vi "Aux TE Controllers Runtime.vi"(8 "Error In":errorcluster, 9 "TE Serial Ports In":T4[](array[typedef]) {"XOFF Char" format="%.0x"; "XON Char" format="%.0x"; "flow control" items=["None"=0, "XON/XOFF"=1, "RTS/CTS"=2, "DTR/DSR"=4]; "stop bits" items=["1.0"=10, "1.5"=15, "2.0"=20]; "data bits" min=5 max=8 step=1; "baud rate" items=["75"=75, "110"=110, "134"=134, "150"=150, "300"=300, "600"=600, "1200"=1200, "1800"=1800, "2400"=2400, "4800"=4800, "7200"=7200, "9600"=9600, "14400"=14400, "19200"=19200, "28800"=28800, "38400"=38400, "56000"=56000, "57600"=57600, "115200"=115200, "128000"=128000, "230400"=230400]; "termination char" format="%.0x"}, 10 "CmdsToWrite":string[](array[string]), 11 "Refs":T1 {"Current Settings"."Pump" items=["Pump 0", "Pump 1", "Pump 2", "Pump 3", "Pump 4", "Pump 5"]; "Current Settings"."Chart X axis Timescale" min=20 max=180 step=1; "Current Settings"."RunTime Mode Settings"."Exp. Gas Tank" items=["0.07", "0.031", "0.877", "1.863", "3.881", "5.790", "7.688", "6.000"]; "Current Settings"."RunTime Mode Settings"."Insp. Gas Tank" items=["0.07", "0.031", "0.877", "1.863", "3.881", "5.790", "7.688", "6.000"]; "Current Settings"."RunTime Mode Settings"."I:E Ratio" max=30 scale=0.0..7.0; "Current Settings"."RunTime Mode Settings"."Resp Rate Brpm" min=0 max=30 format="%.2f"; "Current Settings"."TE#2 Configuration"."Serial Port"."XOFF Char" format="%.0x"; "Current Settings"."TE#2 Configuration"."Serial Port"."XON Char" format="%.0x"; "Current Settings"."TE#2 Configuration"."Serial Port"."flow control" items=["None"=0, "XON/XOFF"=1, "RTS/CTS"=2, "DTR/DSR"=4]; "Current Settings"."TE#2 Configuration"."Serial Port"."stop bits" items=["1.0"=10, "1.5"=15, "2.0"=20]; "Current Settings"."TE#2 Configuration"."Serial Port"."data bits" min=5 max=8 step=1; "Current Settings"."TE#2 Configuration"."Serial Port"."baud rate" items=["75"=75, "110"=110, "134"=134, "150"=150, "300"=300, "600"=600, "1200"=1200, "1800"=1800, "2400"=2400, "4800"=4800, "7200"=7200, "9600"=9600, "14400"=14400, "19200"=19200, "28800"=28800, "38400"=38400, "56000"=56000, "57600"=57600, "115200"=115200, "128000"=128000, "230400"=230400]; "Current Settings"."TE#2 Configuration"."Serial Port"."termination char" format="%.0x"; "Current Settings"."TE#1 Configuration"."Serial Port"."XOFF Char" format="%.0x"; "Current Settings"."TE#1 Configuration"."Serial Port"."XON Char" format="%.0x"; "Current Settings"."TE#1 Configuration"."Serial Port"."flow control" items=["None"=0, "XON/XOFF"=1, "RTS/CTS"=2, "DTR/DSR"=4]; "Current Settings"."TE#1 Configuration"."Serial Port"."stop bits" items=["1.0"=10, "1.5"=15, "2.0"=20]; "Current Settings"."TE#1 Configuration"."Serial Port"."data bits" min=5 max=8 step=1; "Current Settings"."TE#1 Configuration"."Serial Port"."baud rate" items=["75"=75, "110"=110, "134"=134, "150"=150, "300"=300, "600"=600, "1200"=1200, "1800"=1800, "2400"=2400, "4800"=4800, "7200"=7200, "9600"=9600, "14400"=14400, "19200"=19200, "28800"=28800, "38400"=38400, "56000"=56000, "57600"=57600, "115200"=115200, "128000"=128000, "230400"=230400]; "Current Settings"."TE#1 Configuration"."Serial Port"."termination char" format="%.0x"; "Current Settings"."Capnometer Configuration"."Device" items=["None", "TidalWave", "LoFlow / Canary", "Capnogard"]; "Current Settings"."Capnometer Configuration"."Serial Port"."XOFF Char" format="%.0x"; "Current Settings"."Capnometer Configuration"."Serial Port"."XON Char" format="%.0x"; "Current Settings"."Capnometer Configuration"."Serial Port"."flow control" items=["None"=0, "XON/XOFF"=1, "RTS/CTS"=2, "DTR/DSR"=4]; "Current Settings"."Capnometer Configuration"."Serial Port"."stop bits" items=["1.0"=10, "1.5"=15, "2.0"=20]; "Current Settings"."Capnometer Configuration"."Serial Port"."data bits" min=5 max=8 step=1; "Current Settings"."Capnometer Configuration"."Serial Port"."baud rate" items=["75"=75, "110"=110, "134"=134, "150"=150, "300"=300, "600"=600, "1200"=1200, "1800"=1800, "2400"=2400, "4800"=4800, "7200"=7200, "9600"=9600, "14400"=14400, "19200"=19200, "28800"=28800, "38400"=38400, "56000"=56000, "57600"=57600, "115200"=115200, "128000"=128000, "230400"=230400]; "Current Settings"."Capnometer Configuration"."Serial Port"."termination char" format="%.0x"; "Current Settings"."DAQx Settings"."Analog Output Settings (Volts)" format="%#.3g"; "Current Settings"."DAQx Settings"."Duty Cycle" min=10.0 max=90.0 format="%.1g"; "Current Settings"."DAQx Settings"."Frequency" min=20.0 max=200.0; "Current Settings"."DataLogging Settings"."Data File Duration (Minutes)" min=2 max=200 format="%#.2g"; "Current Settings"."Calibration Settings"."Tolerance #2" min=2 max=4096; "Current Settings"."Calibration Settings"."Cal. Average" min=2 max=4096; "Current Settings"."Test Settings"."Test Sensor ID" items=["(select)", "RB", "YC", "", "Other"]}) -> (0 "Error Out":errorcluster, 1 "Read Array":string[][](array[string]), 2 "ReadData":sgl[][](array[numeric]) format="%.2g", 3 "TE Serial Ports Out":T4[](array[typedef]) {"XOFF Char" format="%.0x"; "XON Char" format="%.0x"; "flow control" items=["None"=0, "XON/XOFF"=1, "RTS/CTS"=2, "DTR/DSR"=4]; "stop bits" items=["1.0"=10, "1.5"=15, "2.0"=20]; "data bits" min=5 max=8 step=1; "baud rate" items=["75"=75, "110"=110, "134"=134, "150"=150, "300"=300, "600"=600, "1200"=1200, "1800"=1800, "2400"=2400, "4800"=4800, "7200"=7200, "9600"=9600, "14400"=14400, "19200"=19200, "28800"=28800, "38400"=38400, "56000"=56000, "57600"=57600, "115200"=115200, "128000"=128000, "230400"=230400]; "termination char" format="%.0x"}, 4 "TE Bytes Read":i16[][](array[numeric]), 5 "Set Point Good":bool, 6 "TE Data":sgl[][](array[numeric]), 7 "Set Point Disabled":bool)   [LabVIEW 2016]
uses:
  Controls/Serial Visa Control.ctl
  Controls/DAQ Needed.ctl
  Controls/Processed Variables.ctl
  Controls/AirPump Controls.ctl
  Controls/IE Ratio knob.ctl
  Controls/UI Settings.ctl
  Controls/Aux CO2 Control.ctl
  Controls/Aux CO2 Selector.ctl
  Controls/Aux TE Control.ctl
  Controls/Queues And Others.ctl
  Controls/SerialPortControl.ctl
  Miscellaneous/Globals.vi
panel:
  out "after substring":string
  out "appended array":string[][](array[string])
  out "subarray":dbl[](array[numeric])
  out "size(s)":i32[](array[numeric])
  # "Note: Setting Brpm to zero will\ndisable Insp / Exp digital output."
  # "mmHg"
  # "pts"
  # "tolerance"
  # "AN5 (Temp 1)"
  # "AN6 (Temp 2)"
  # "AN7 (Temp 3)"
  # "AN8 (T FET)"
  # "AN0 (T POT)"
  # "Tref (Set Pt))"
  # "(Spare)"
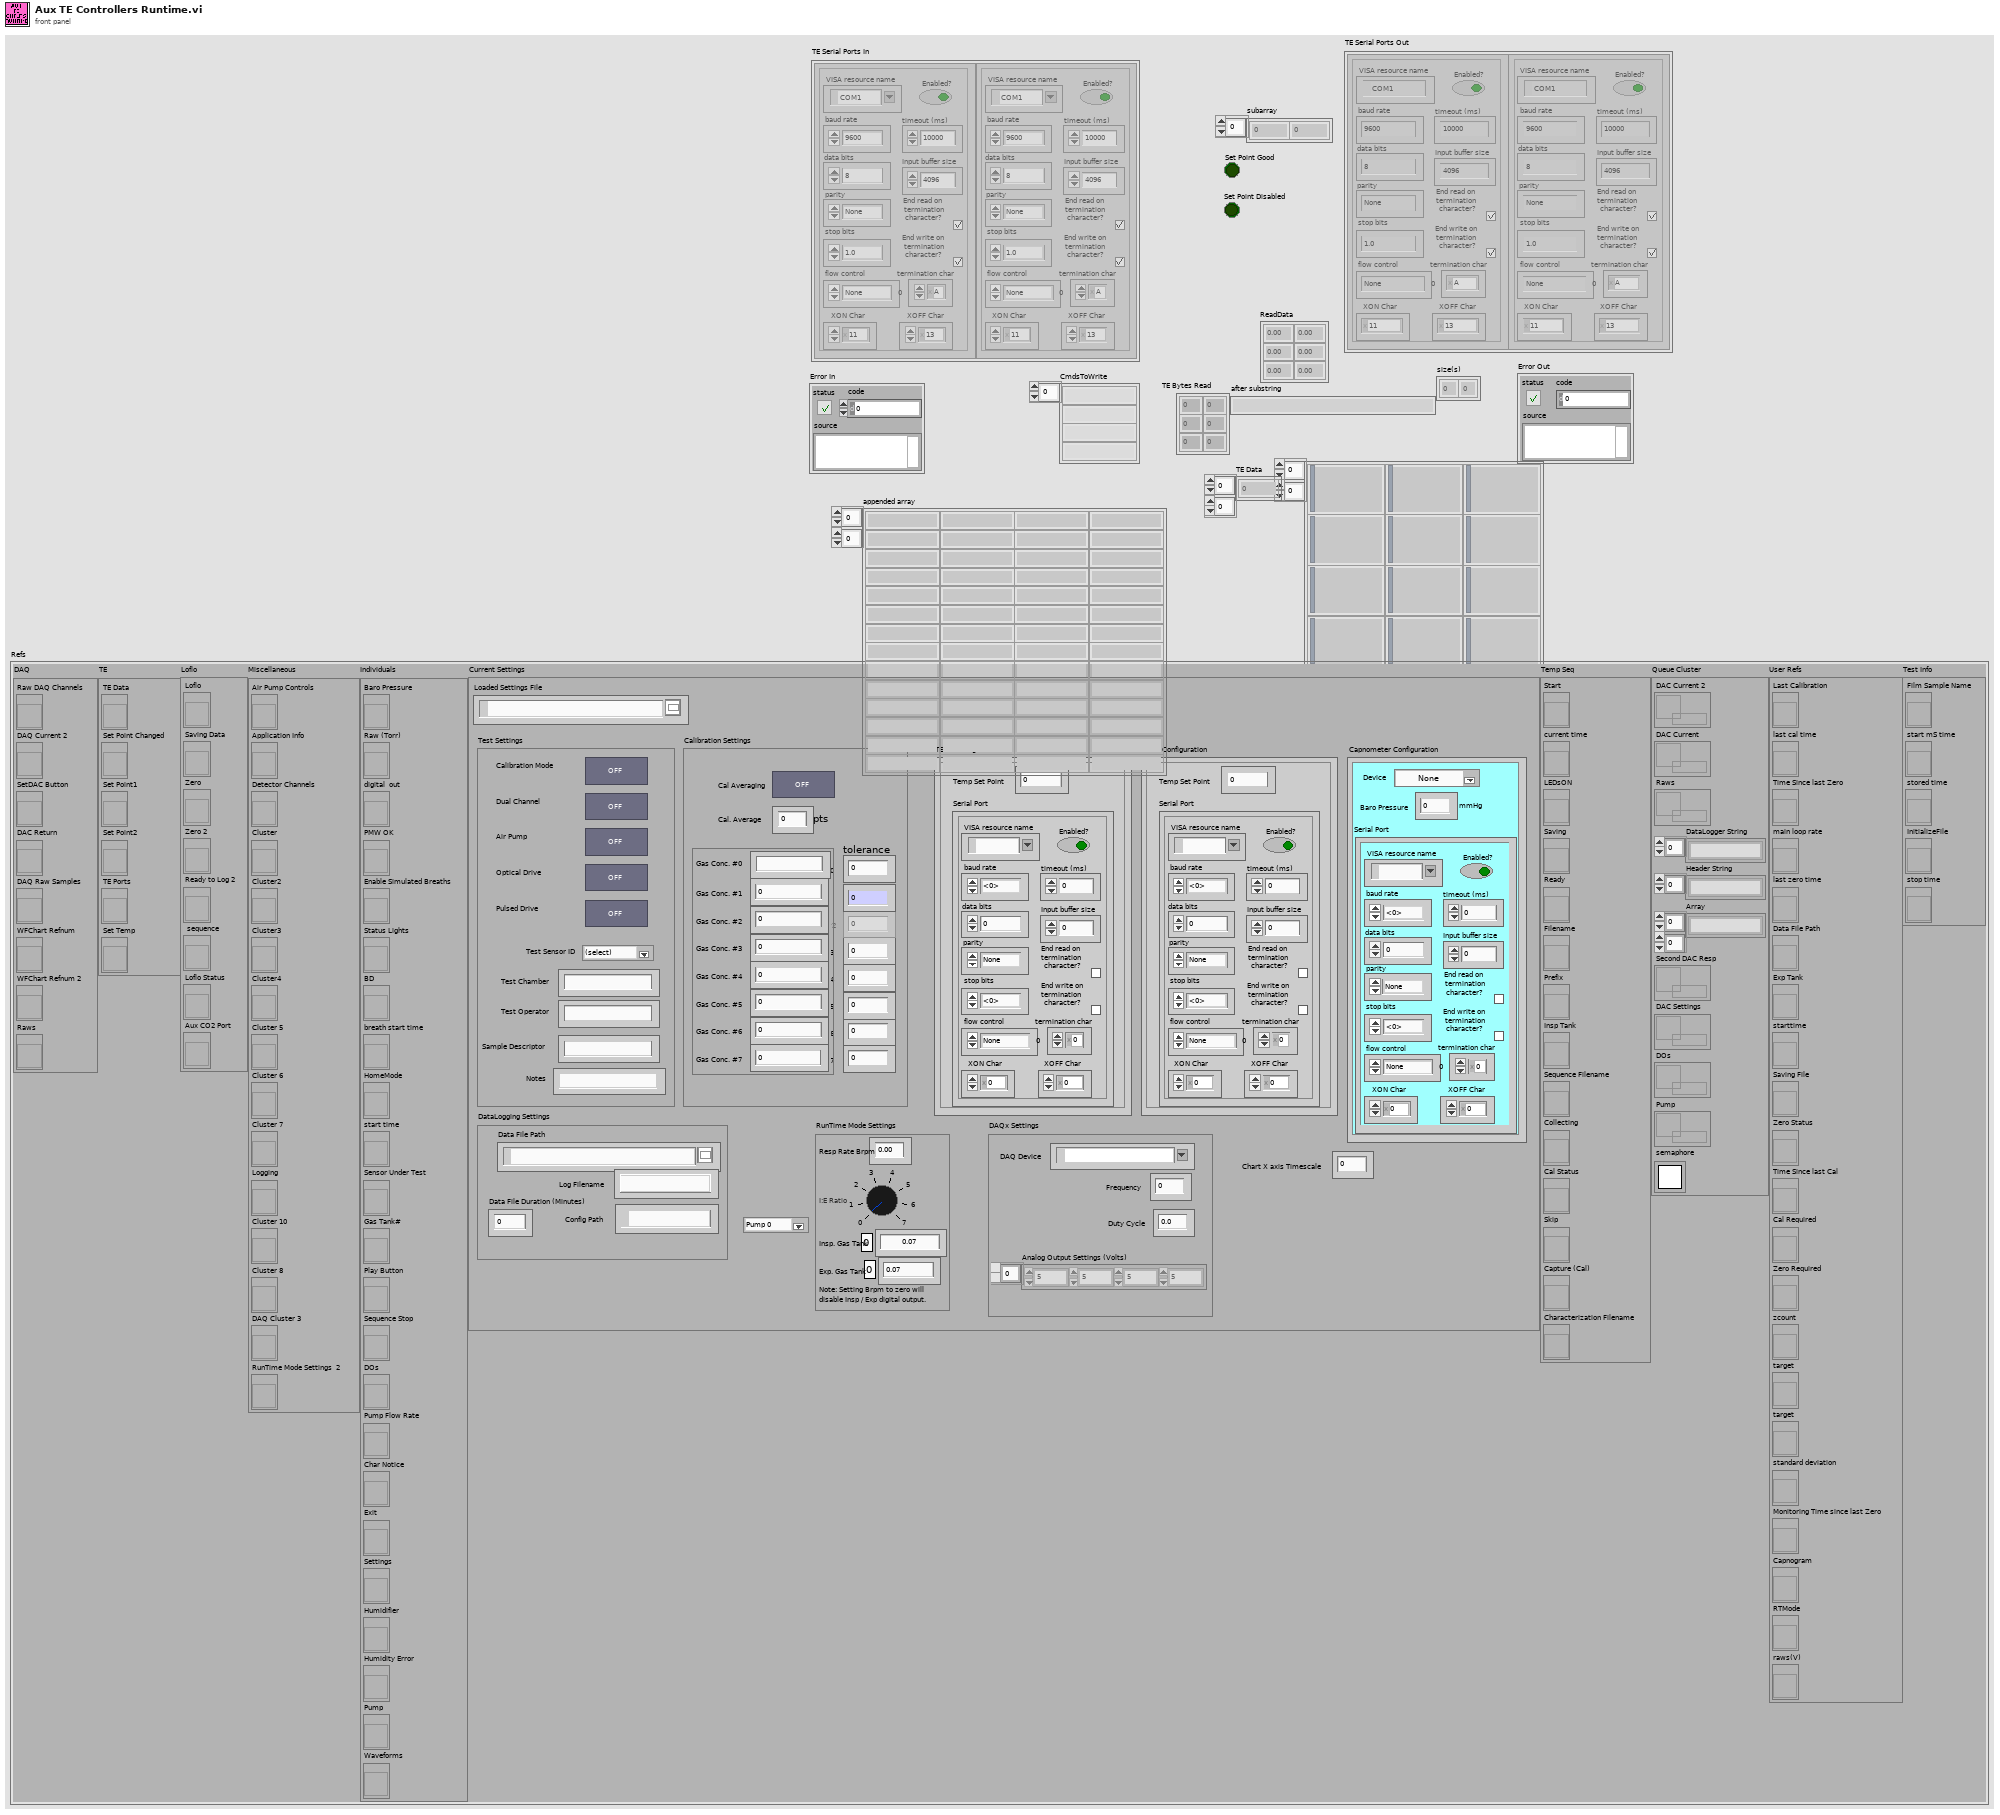
[diagram p1: front panel]
types:
  T1 = typedef "DAQ Needed.ctl" = cluster{"DAQ":cluster{"Raw DAQ Channels":refnum<vi>, "DAQ Current 2":refnum<vi>, "SetDAC Button":refnum<vi>, "DAC Return":refnum<vi>, "DAQ Raw Samples":refnum<vi>, "WFChart Refnum":refnum<vi>, "WFChart Refnum 2":refnum<vi>, "Raws":refnum<vi>}, "TE":cluster{"TE Data":refnum<vi>, "Set Point Changed":refnum<vi>, "Set Point1":refnum<vi>, "Set Point2":refnum<vi>, "TE Ports":refnum<vi>, "Set Temp":refnum<vi>}, "Loflo":cluster{"Loflo":refnum<vi>, "Saving Data":refnum<vi>, "Zero":refnum<vi>, "Zero 2":refnum<vi>, "Ready to Log 2":refnum<vi>, " sequence":refnum<vi>, "Loflo Status ":refnum<vi>, "Aux CO2 Port":refnum<vi>}, "Miscellaneous":cluster{"Air Pump Controls":refnum<vi>, "Application Info":refnum<vi>, "Detector Channels ":refnum<vi>, "Cluster":refnum<vi>, "Cluster2":refnum<vi>, "Cluster3":refnum<vi>, "Cluster4":refnum<vi>, "Cluster 5":refnum<vi>, "Cluster 6":refnum<vi>, "Cluster 7":refnum<vi>, "Logging":refnum<vi>, "Cluster 10":refnum<vi>, "Cluster 8":refnum<vi>, "DAQ Cluster 3":refnum<vi>, "RunTime Mode Settings  2":refnum<vi>}, "Individuals":cluster{"Baro Pressure":refnum<vi>, "Raw (Torr)":refnum<vi>, "digital  out":refnum<vi>, "PMW OK":refnum<vi>, "Enable Simulated Breaths":refnum<vi>, "Status Lights":refnum<vi>, "BD":refnum<vi>, "breath start time":refnum<vi>, "HomeMode":refnum<vi>, "start time":refnum<vi>, "Sensor Under Test":refnum<vi>, "Gas Tank#":refnum<vi>, "Play Button":refnum<vi>, "Sequence Stop":refnum<vi>, "DOs":refnum<vi>, "Pump Flow Rate":refnum<vi>, "Char Notice":refnum<vi>, "Exit":refnum<vi>, "Settings":refnum<vi>, "Humidifier":refnum<vi>, "Humidity Error":refnum<vi>, "Pump":refnum<vi>, "Waveforms":refnum<vi>}, "Current Settings":T2, "Temp Seq":cluster{"Start":refnum<vi>, "current time":refnum<vi>, "LEDsON":refnum<vi>, "Saving":refnum<vi>, "Ready":refnum<vi>, "Filename":refnum<vi>, "Prefix":refnum<vi>, "Insp Tank":refnum<vi>, "Sequence Filename":refnum<vi>, "Collecting":refnum<vi>, "Cal Status":refnum<vi>, "Skip":refnum<vi>, "Capture (Cal)":refnum<vi>, "Characterization Filename":refnum<vi>}, "Queue Cluster":T7, "User Refs":cluster{"Last Calibration":refnum<vi>, "last cal time":refnum<vi>, "Time Since last Zero":refnum<vi>, "main loop rate":refnum<vi>, "last zero time":refnum<vi>, "Data File Path":refnum<vi>, "Exp Tank":refnum<vi>, "starttime":refnum<vi>, "Saving File":refnum<vi>, "Zero Status":refnum<vi>, "Time Since last Cal":refnum<vi>, "Cal Required":refnum<vi>, "Zero Required":refnum<vi>, "zcount":refnum<vi>, "target":refnum<vi>, "target":refnum<vi>, "standard deviation":refnum<vi>, "Monitoring Time since last Zero":refnum<vi>, "Capnogram":refnum<vi>, "RTMode":refnum<vi>, "raws(V)":refnum<vi>}, "Test Info":cluster{"Film Sample Name":refnum<vi>, "start mS time":refnum<vi>, "stored time":refnum<vi>, "InitializeFile":refnum<vi>, "stop time":refnum<vi>}}
  T2 = typedef "UI Settings.ctl" = cluster{"Loaded Settings File":path, "Test Settings":cluster{"Dual Channel":bool, "Air Pump":bool, "Optical Drive":bool, "Pulsed Drive":bool, "Calibration Mode":bool, "Test Sensor ID":u16, "Test Chamber":string, "Test Operator":string, "Sample Descriptor":string, "Notes":string}, "Calibration Settings":cluster{"Cal. Average":u16, "Cal Averaging":bool, "Tolerance #0":sgl, "Tolerance #7":sgl, "Tolerance #6":sgl, "Tolerance #5":sgl, "Tolerance #4":sgl, "Tolerance #3":sgl, "Tolerance #2":sgl, "Tolerance #1":sgl, "Gas Tank Settings":cluster{"Gas Conc. #0":string, "Gas Conc. #1":sgl, "Gas Conc. #2":sgl, "Gas Conc. #3":sgl, "Gas Conc. #4":sgl, "Gas Conc. #5":sgl, "Gas Conc. #6":sgl, "Gas Conc. #7":sgl}}, "DataLogging Settings":cluster{"Data File Path":path, "Data File Duration (Minutes)":sgl, "Log Filename":string, "Config Path":path}, "DAQx Settings":cluster{"DAQ Device":tag, "Frequency":dbl, "Duty Cycle":dbl, "Analog Output Settings (Volts)":sgl[]}, "Capnometer Configuration":T3, "TE#1 Configuration":T6, "TE#2 Configuration":T6, "RunTime Mode Settings ":cluster{"Resp Rate Brpm ":sgl, "I:E Ratio":u8, "Insp. Gas Tank":u16, "Exp. Gas Tank":u16}, "Chart X axis Timescale":u16, "Pump":u16}
  T3 = typedef "Aux CO2 Control.ctl" = cluster{"Serial Port":T4, "Baro Pressure":u32, "Device":T5}
  T4 = typedef "Serial Visa Control.ctl" = cluster{"termination char":u8, "End read on termination character?":bool, "Enabled?":bool, "VISA resource name":refnum<visa-resource-name>, "baud rate":u32, "data bits":u16, "parity":enum16{"None", "Odd", "Even", "Mark", "Space"}, "stop bits":u16, "flow control":u16, "timeout (ms)":u32, "Input buffer size":u32, "End write on termination character?":bool, "XON Char":u8, "XOFF Char":u8}
  T5 = typedef "Aux CO2 Selector.ctl" = u16
  T6 = typedef "Aux TE Control.ctl" = cluster{"Temp Set Point":sgl, "Serial Port":T4}
  T7 = typedef "Queues And Others.ctl" = cluster{"DAC Current 2":refnum<queue>, "DAC Current":refnum<queue>, "Raws":refnum<queue>, "DataLogger String":string[], "Header String":string[], "Array":string[][], "Second DAC Resp":refnum<queue>, "DAC Settings":refnum<queue>, "DOs":refnum<queue>, "Pump":refnum<queue>, "semaphore":T8}
  T8 = typedef "Semaphore RefNum" = refnum<k1>
  T9 = typedef "SerialPortControl.ctl" = enum16{"Initialize", "Write Data", "Read Data", "Close Port"}
  T10 = cluster{"Ref CO2":sgl, "Humidity":sgl, "TE #1":sgl, "TE #2":sgl, " Film `C":dbl, "Bath `C":dbl, " Det. `C":dbl, " Ambient":dbl, " Chamber C ":dbl}
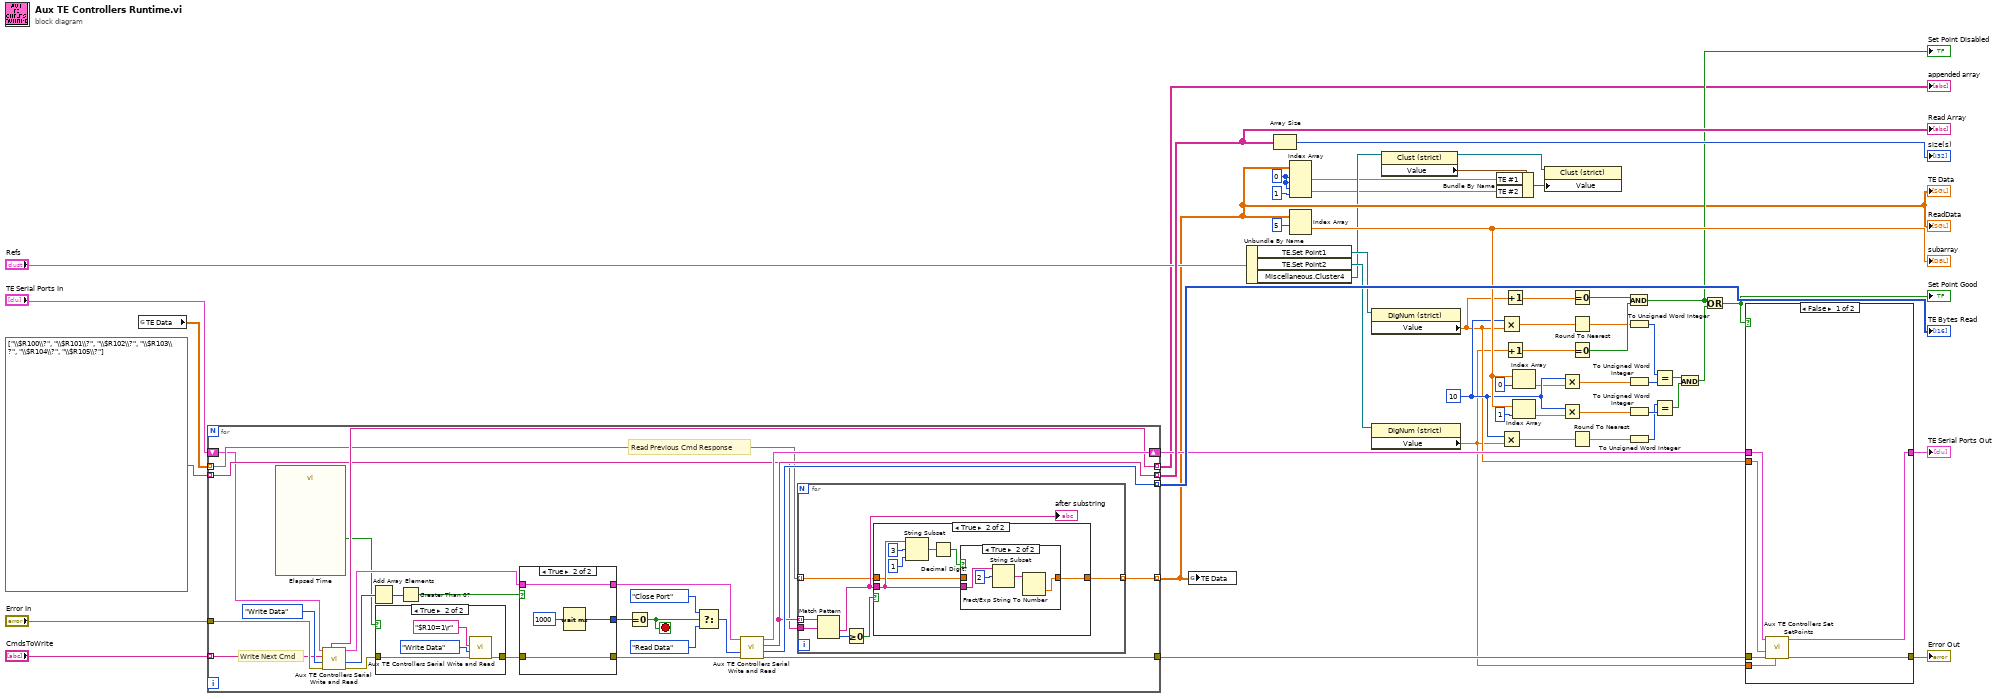
[diagram p0: block diagram]
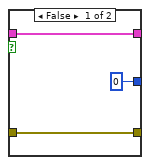
[diagram p6: hidden frame]
diagram:
  w16 = 0 ("index (row)")
  w40 = 10
  n1 = global read "Globals.vi" "TE Data"() -> (w10:sgl[][])
  n2 = for {
    tunnel: [w76] -> w33
    tunnel: "Error In" -> [w78]
    tunnel: [w75] -> w51 mode=indexing
    tunnel: "CmdsToWrite" -> [w61] mode=indexing
    tunnel: [w62] -> w52 mode=indexing
    tunnel: [w60] -> w9 mode=indexing
    tunnel: [w63] -> w11 mode=indexing
    tunnel: string[] ["\\$R100\\?", "\\$R101\\?", "\\$R102\\?", "\\$R103\\?", "\\$R104\\?", "\\$R105\\?"] ("CmdsToWrite") -> [w59] mode=indexing
    tunnel: w10 -> [w58] mode=indexing
    shift-right: [w77] -> w35
    shift-left: "TE Serial Ports In" -> [w57]
    stop <- w64 stop-if-true
    # "Read Previous Cmd Response"
    # "Write Next Cmd"
    n3 = call "Elapsed Time"() -> ("Time has Elapsed"=w56:bool)  [unwired: 12 in, 7 out]
    n4 = call "Aux TE Controllers Serial Write and Read.vi"("error in"=w78, "Action"=SerialPortControl."Write Data", "string to write"=w61, "TE Controller Serial Ports In"=w57) -> ("Error Out"=w55:errorcluster, "#Bytes R/W"=w69:i16[], "TE Controller Serial Ports Out"=w74:T4[], "appended array"=w63:string[])  [unwired: 1 in, 1 out]
    n5 = Add Array Elements(numeric array=w69) -> (sum=w71:i16)
    n6 = case shown="True" w56 {
      tunnel: w55 -> [w80 w82]
      tunnel: [w80 w81] -> w54
      frame False {
      }
      frame True {
        n7 = call "Aux TE Controllers Serial Write and Read.vi"("error in"=w82, "Action"=SerialPortControl."Write Data", "string to write"="$R10=1\r") -> ("Error Out"=w81:errorcluster)  [unwired: 2 in, 4 out]
      }
    }
    n8 = Greater Than 0?(x=w71) -> (x > 0?=w70:bool)
    n9 = case shown="True" w70 {
      tunnel: [w106 w111] -> w73
      tunnel: w74 -> [w106 w111]
      tunnel: [w107 w110] -> w72
      tunnel: w54 -> [w107 w110]
      tunnel: [u32 0 ("millisecond timer value") w108] -> w68
      frame False {
      }
      frame True {
        n10 = Wait (ms)(milliseconds to wait=i16 1000 ("y")) -> (millisecond timer value=w108:u32)
      }
    }
    n11 = Equal To 0?(x=w68) -> (x = 0?=w64:bool)
    n12 = Select(t=SerialPortControl."Close Port" ("Action"), s=w64, f=SerialPortControl."Read Data" ("Action")) -> (s? t:f=w67:T9)
    n13 = call "Aux TE Controllers Serial Write and Read.vi"("error in"=w72, "Action"=w67, "TE Controller Serial Ports In"=w73) -> ("Error Out"=w76:errorcluster, "#Bytes R/W"=w75:i16[], "Data Read"=w62:string[], "TE Controller Serial Ports Out"=w77:T4[])  [unwired: 2 in, 1 out]
    n14 = for {
      tunnel: w62 -> [w91] mode=indexing
      tunnel: w59 -> [w90]
      tunnel: [w88] -> w60 mode=indexing
      tunnel: w58 -> [w87] mode=indexing
      n15 = Match Pattern(string=w91, regular expression=w90) -> (after substring=w89:string, offset past match=w86:i32)  [unwired: 1 in, 2 out]
      "after substring" <- w89
      n16 = Greater Or Equal To 0?(x=w86) -> (x >= 0?=w85:bool)
      n17 = case shown="True" w85 {
        tunnel: w89 -> [_ w94]
        tunnel: [w92 w99] -> w88
        tunnel: w87 -> [w92 w93]
        frame False {
        }
        frame True {
          n18 = String Subset(string=w94, offset (0)=3, length (rest)=1 ("length (rest)")) -> (substring=w96:string)
          n19 = Decimal Digit?(1:w96) -> (0:w95:bool)
          n20 = case shown="True" w95 {
            tunnel: [w100 w104] -> w99
            tunnel: w94 -> [_ w102]
            tunnel: w93 -> [w100 _]
            frame False {
            }
            frame True {
              n21 = String Subset(string=w102, offset (0)=2) -> (substring=w101:string)  [unwired: 1 in]
              n22 = Fract/Exp String To Number(string=w101) -> (number=w104:dbl)  [unwired: 3 in, 1 out]
            }
          }
        }
      }
    }
  }
  "TE Bytes Read" <- w51
  "Read Array" <- w52
  "ReadData" <- w9
  "TE Data" <- w9
  "appended array" <- w11
  n23 = global write "Globals.vi" "TE Data"(w9) -> ()
  n24 = Unbundle By Name("Refs") -> ("TE.Set Point1"=w13:refnum<vi>, "TE.Set Point2"=w12:refnum<vi>, "Miscellaneous.Cluster4"=w6:refnum<vi>)
  n25 = Array Size(array=w52) -> (size(s)=→"size(s)":i32[])
  n26 = Index Array(array=w9, index (row) #1=w16, index (col) #1=w16, index (row) #2=w16, index (col) #2=1 ("disabled index (col)")) -> (element #1=w2:dbl, element #2=w1:dbl)
  n27 = Index Array(array=w9, index (row)=5) -> (element=w45:dbl[])  [unwired: 1 in]
  "subarray" <- w45
  n28 = property class="DigNum (strict)"(reference=w13) -> ("Value"=w18:sgl)  [unwired: 1 in, 2 out]
  n29 = property class="DigNum (strict)"(reference=w12) -> ("Value"=w17:sgl)  [unwired: 1 in, 2 out]
  n30 = property class="Clust (strict)"(reference=w6) -> (reference out=w5:refnum<vi>, "Value"=w4:T10)  [unwired: 1 in, 1 out]
  n31 = Bundle By Name(cluster=w4, "TE #1"=w2, "TE #2"=w1) -> (w3:T10)
  n32 = Multiply(x=w40, y=w18) -> (x*y=w21:sgl)
  n33 = Multiply(x=w40, y=w17) -> (x*y=w23:sgl)
  n34 = Increment(x=w18) -> (x+1=w31:sgl)
  n35 = Increment(x=w17) -> (x+1=w30:sgl)
  n36 = Index Array(array=w45, index=0) -> (element=w39:dbl)
  n37 = Index Array(array=w45, index=1) -> (element=w41:dbl)
  n38 = property class="Clust (strict)"(reference=w5, "Value"=w3) -> ()  [unwired: 1 in, 2 out]
  n39 = Multiply(x=w40, y=w39) -> (x*y=w22:dbl)
  n40 = Multiply(x=w40, y=w41) -> (x*y=w24:dbl)
  n41 = Equal To 0?(x=w31) -> (x = 0?=w28:bool)
  n42 = Round To Nearest(number=w21) -> (nearest integer value=w20:sgl)
  n43 = Equal To 0?(x=w30) -> (x = 0?=w29:bool)
  n44 = Round To Nearest(number=w23) -> (nearest integer value=w19:sgl)
  n45 = And(x=w28, y=w29) -> (x .and. y?=w25:bool)
  "Set Point Disabled" <- w25
  n46 = To Unsigned Word Integer(number=w20) -> (unsigned 16bit integer=w36:u16)
  n47 = To Unsigned Word Integer(number=w22) -> (unsigned 16bit integer=w37:u16)
  n48 = To Unsigned Word Integer(number=w24) -> (unsigned 16bit integer=w42:u16)
  n49 = To Unsigned Word Integer(number=w19) -> (unsigned 16bit integer=w38:u16)
  n50 = Equal?(x=w36, y=w37) -> (x = y?=w43:bool)
  n51 = Equal?(x=w38, y=w42) -> (x = y?=w44:bool)
  n52 = And(x=w43, y=w44) -> (x .and. y?=w27:bool)
  n53 = Or(x=w25, y=w27) -> (x .or. y?=w26:bool)
  "Set Point Good" <- w26
  n54 = case shown="False" w26 {
    tunnel: [w114 w119] -> w34
    tunnel: w35 -> [w117 w119]
    tunnel: [w115 w118] -> w32
    tunnel: w33 -> [w116 w118]
    tunnel: w18 -> [w113 _]
    tunnel: w17 -> [w112 _]
    frame False {
      n55 = call "Aux TE Controllers Set SetPoints.vi"("Set Point2"=w112, "Error In"=w116, "Set Point1"=w113, "TE Serial Ports In"=w117) -> ("Error Out"=w115:errorcluster, "TE Serial Ports Out"=w114:T4[])  [unwired: 5 in, 1 out]
    }
    frame True {
    }
  }
  "TE Serial Ports Out" <- w34
  "Error Out" <- w32
